vi "daqmx_digital_1ch1line.vi"() -> ()   [LabVIEW 2019]
uses:
  <vilib>/DAQmx/read.llb/DAQmx Read (Digital U8 1Chan 1Samp).vi
  <vilib>/DAQmx/create/channels.llb/DAQmx Create Channel (DI-Digital Input).vi
  <vilib>/DAQmx/configure/task.llb/DAQmx Configure Logging (TDMS).vi
  <vilib>/DAQmx/miscellaneous.llb/DAQmx Fill In Error Info.vi
panel:
  in  "DAQmx Physical Channel":tag="PXI1Slot7/port0/line0"
  out "Error Out":errorcluster
  in  "TDMS File":path=path "C:/Python/projects/nitdms/tests/tdms_files/daqmx_digital_1ch1line.tdms"
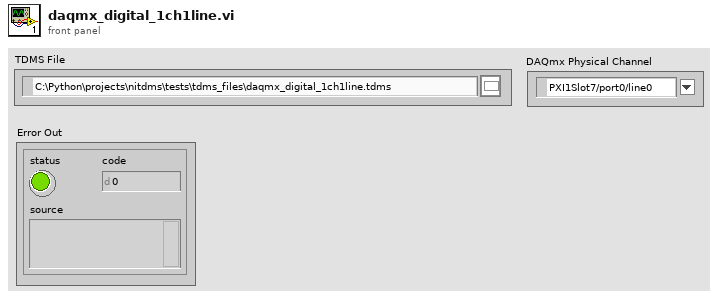
[diagram p1: front panel]
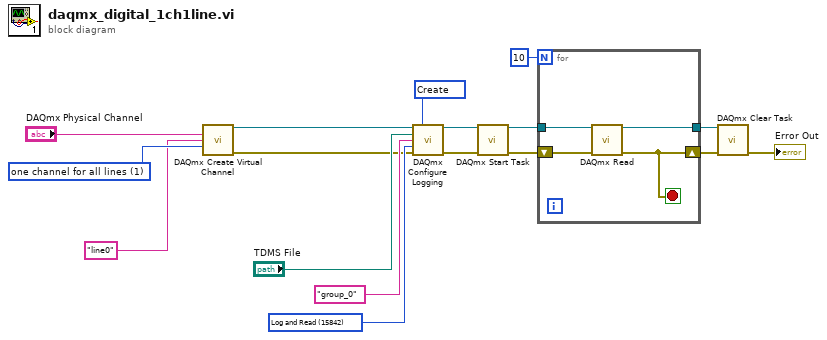
[diagram p0: block diagram]
diagram:
  w2 = 1 items=["one channel for each line", "one channel for all lines"] ("line grouping")
  w13 = 15842 items=["Off"=10231, "Log"=15844, "Log and Read"=15842] ("logging mode")
  w15 = 15848 items=["Open"=10437, "Open or Create"=15846, "Create or Replace"=15847, "Create"=15848] ("operation")
  n1 = call-poly <vilib>:"DAQmx Create Virtual Channel.vi"("lines"="DAQmx Physical Channel", "name to assign"="line0", "line grouping"=w2) -> ("task out"=w8:refnum<k21>, "error out"=w9:errorcluster)  [unwired: 11 in]
  n2 = call-poly <vilib>:"DAQmx Configure Logging.vi"("task/channels in"=w8, "operation"=w15, "file path"="TDMS File", "group name"="group_0", "logging mode"=w13, "error in"=w9) -> ("task out"=w11:refnum<k21>, "error out"=w12:errorcluster)  [unwired: 8 in]
  n3 = call <vilib>:"DAQmx Start Task.vi"("task/channels in"=w11, "error in"=w12) -> ("task out"=w6:refnum<k21>, "error out"=w7:errorcluster)  [unwired: 12 in]
  n4 = for {
    N: 10 -> [_]
    shift-right: [w18] -> w5
    shift-left: w7 -> [w21]
    tunnel: w6 -> [w20]
    tunnel: [w19] -> w3
    stop <- w18 stop-if-true
    n5 = call-poly <vilib>:"DAQmx Read.vi"("task/channels in"=w20, "error in"=w21) -> ("task out"=w19:refnum<k21>, "error out"=w18:errorcluster)  [unwired: 11 in, 1 out]
  }
  n6 = call <vilib>:"DAQmx Clear Task.vi"("task in"=w3, "error in"=w5) -> ("error out"=→"Error Out":errorcluster)  [unwired: 13 in]
